vi "Wirte Signal.vi"(8 "error in (no error)":errorcluster, 9 "Signal Write":dbl, 10 "Tx Signal In":string="GIP_TestMode.GIP_TestModeFlag", 11 "CAN in":refnum<class "CAN.lvclass">) -> (0 "error out":errorcluster, 3 "CAN out":refnum<class "CAN.lvclass">)   [LabVIEW 2019, in "CAN.lvclass"]
uses:
  CAN.lvclass
  CAN.lvclass/CAN.ctl
  <vilib>/JDP Science/JSONtext/Next JSON Value.vi
  <vilib>/JDP Science/JSONtext/String Subset.vi
  <vilib>/JDP Science/JSONtext/Parsing/Advance past next JSON Value (inlined COPY).vi
  <vilib>/JDP Science/JSONtext/Parsing/Advance past whitespace.vi
  <vilib>/JDP Science/JSONtext/Parsing/Advance past String.vi
  <vilib>/JDP Science/JSONtext/Parsing/Advance past Number.vi
  <vilib>/JDP Science/JSONtext/Parsing/Advance past Line Ending.vi
  <vilib>/JDP Science/JSONtext/Parsing/Parse Full Path or Item Name.vi
  <vilib>/JDP Science/JSONtext/Parsing/Advance past Array.vi
  <vilib>/JDP Science/JSONtext/Parsing/Advance past Object.vi
  <vilib>/JDP Science/JSONtext/support/Error Cluster From Code.vi
  <vilib>/JDP Science/JSONtext/Offset/Find Item Locations by Path.vi
  <vilib>/xnet/xnet.llb/XNET Write (Signal Single-point).vi
  <vilib>/JDP Science/JSONtext/JSONtext.lvlib
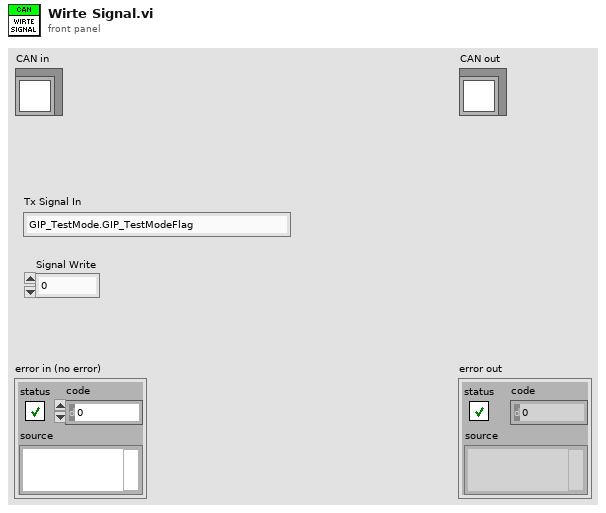
[diagram p1: front panel]
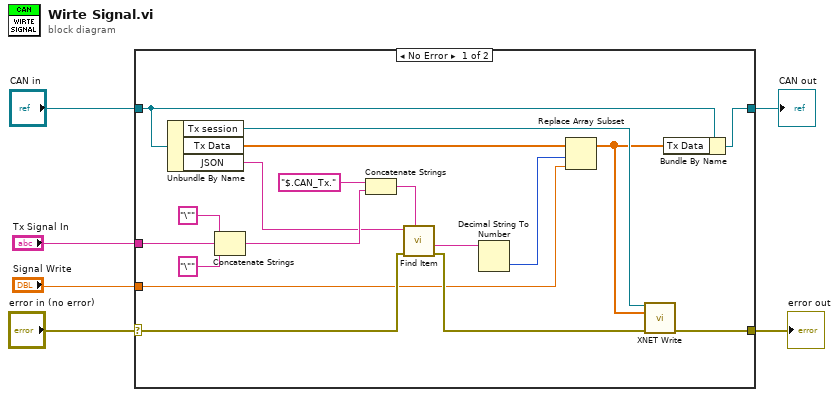
[diagram p0: block diagram]
diagram:
  n1 = case shown="No Error" "error in (no error)" {
    selector: "error in (no error)" -> [w14 w26]
    tunnel: [w13 w26] -> w5
    tunnel: [w8 w25] -> w3
    tunnel: "CAN in" -> [w9 w25]
    tunnel: "Tx Signal In" -> [w12 _]
    tunnel: "Signal Write" -> [w11 _]
    frame No Error {
      n2 = Unbundle By Name(w9) -> ("Tx session"=w10:refnum<k21>, "Tx Data"=w21:dbl[], "JSON"=w18:string)
      n3 = Concatenate Strings("\"" ("string"), w12, "\"" ("string")) -> (w23:string)
      n4 = Concatenate Strings("$.CAN_Tx." ("$Path or Item Name"), w23) -> (w17:string)
      n5 = call <vilib>:"Find Item.vi"("$Path or Item Name"=w17, "error in (no error)"=w14, "JSON"=w18) -> ("error out"=w20:errorcluster, "<JSON>"=w15:string)  [unwired: 5 in, 2 out]
      n6 = Decimal String To Number(string=w15) -> (number=w19:i32)  [unwired: 2 in, 1 out]
      n7 = Replace Array Subset(array=w21, new element=w11, index=w19) -> (w7:dbl[])
      n8 = call-poly <vilib>:"XNET Write.vi"("session in"=w10, "data"=w7, "error in (no error)"=w20) -> ("error out"=w13:errorcluster)  [unwired: 12 out]
      n9 = Bundle By Name(cluster=w9, "Tx Data"=w7) -> (w8:refnum<class "CAN.lvclass">)
    }
    frame Error {
    }
  }
  "error out" <- w5
  "CAN out" <- w3
